vi "Load DSF Configuration File.vi"(8 "error in (no error)":errorcluster, 10 "Path":path, 11 "Application Refs":T1) -> (0 "error out":errorcluster, 3 "Application Data out":T1)   [LabVIEW 2017, in "DSF Mini Explorer.lvlib"]
uses:
  DSF Mini Explorer.lvlib
  Application Data.ctl
  VeriStand/Data Sharing Custom Device/Source/DSF Core.lvlibp/Classes/Configuration/Configuration Session.lvclass
  View Mode.ctl
panel:
  # "App\nData"
  # "App\nData"
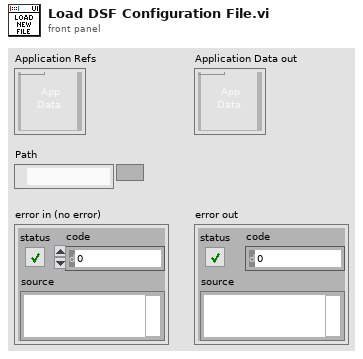
[diagram p1: front panel]
types:
  T1 = typedef "DSF Mini Explorer.lvlib/Application Data.ctl" = cluster{"Item Tree Control":refnum<vi>, "Value Tree Control":refnum<vi>, "DSF Refnum":refnum<class "Configuration Session.lvclass">, "Top-Level VI":refnum<vi>, "View State":T2, "menu reference":refnum<k9>}
  T2 = typedef "DSF Mini Explorer.lvlib/View Mode.ctl" = enum16{"Tree", "List"}
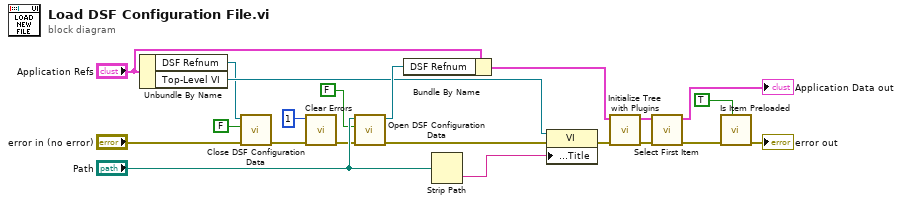
[diagram p0: block diagram]
diagram:
  n1 = Unbundle By Name("Application Refs") -> ("DSF Refnum"=w11:refnum<class "Configuration Session.lvclass">, "Top-Level VI"=w14:refnum<vi>)
  n2 = call "Close DSF Configuration Data.vi"("error in (no error)"="error in (no error)", "write file if changed (T)"=FALSE, "Configuration Session"=w11) -> ("error out"=w12:errorcluster)  [unwired: 7 in, 1 out]
  n3 = call <vilib>:"Clear Errors.vi"("error in (no error)"=w12, "specific error code to clear (0: all)"=1) -> ("error out"=w9:errorcluster)  [unwired: 4 in, 1 out]
  n4 = call "Open DSF Configuration Data.vi"("error in (no error)"=w9, "create file if necessary (T)"=FALSE, "dsf configuration file path"="Path") -> ("error out"=w2:errorcluster, "Configuration Session"=w17:refnum<class "Configuration Session.lvclass">)  [unwired: 4 in, 3 out]
  n5 = Bundle By Name(cluster="Application Refs", "DSF Refnum"=w17) -> (w16:T1)
  n6 = Strip Path(path="Path") -> (name=w1:string)  [unwired: 1 out]
  n7 = property class="VI"(reference=w14, error in=w2, "Front Panel.Title"=w1) -> (error out=w21:errorcluster)  [unwired: 1 out]
  n8 = call "Initialize Tree with Plugins.vi"("error in (no error)"=w21, "Application Data in"=w16) -> ("error out"=w6:errorcluster, "Application Data out"=w7:T1)  [unwired: 8 in]
  n9 = call "Select First Item.vi"("error in (no error)"=w6, "Application Data in"=w7) -> ("error out"=w5:errorcluster, "Application Data out"=→"Application Data out":T1)  [unwired: 8 in]
  n10 = call "Is Item Preloaded"("clear entries"=TRUE, "error in (no error)"=w5) -> ("error out"=→"error out":errorcluster)  [unwired: 7 in, 2 out]
